vi "LogError.vi"(0 "Core In":refnum<class "Core.lvclass">, 11 "Error In":errorcluster {"Code" format="%.0x"}) -> (4 "Core Out":refnum<class "Core.lvclass">, 15 "Error Out":errorcluster {"Code" format="%.0x"})   [LabVIEW 2020, in "Core.lvlib" / "Core.lvclass"]
doc: "Logs error information from general error cluster and handles error codes based on the following conditions:\n- General errors (500,000 to 510,000)\n- Critical errors (510,001 to 520,000)\n- Fatal errors (520,001 to 530,000)"
uses:
  Core.lvclass
  Core.lvclass/Core.ctl
panel:
  # "/* Inputs */"
  # "/* Locals */"
  # "/* Outputs */"
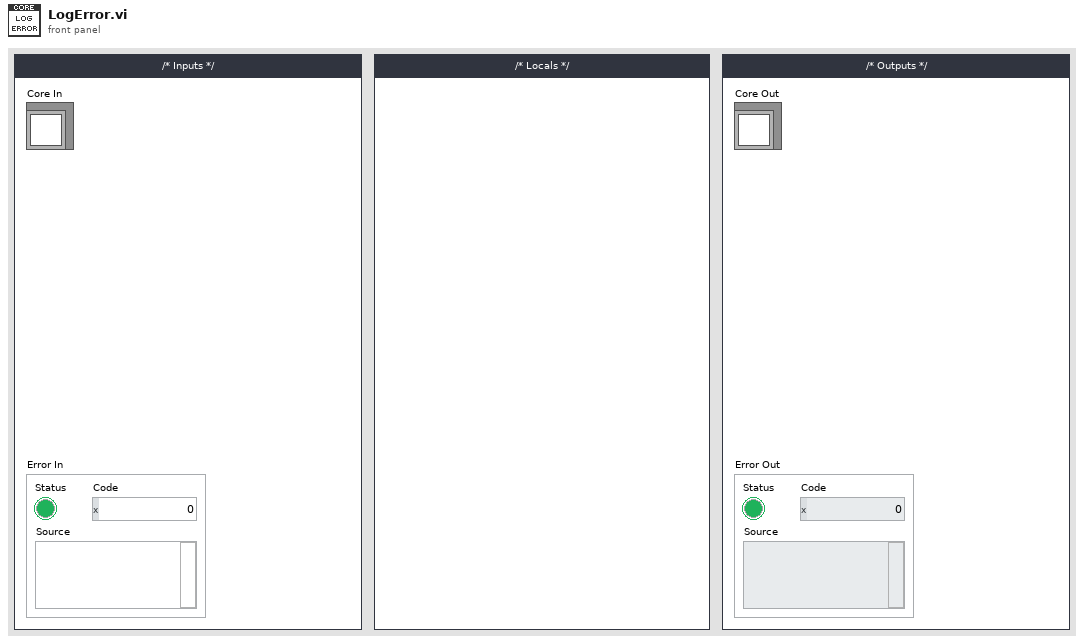
[diagram p1: front panel]
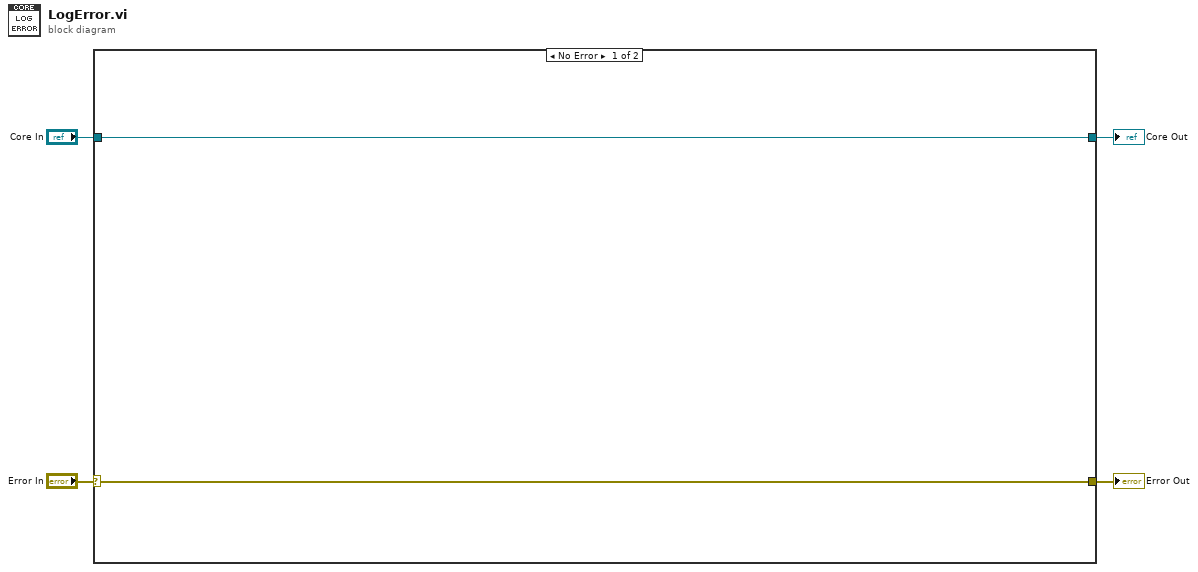
[diagram p0: block diagram]
diagram:
  n1 = case shown="No Error" "Error In" {
    selector: "Error In" -> [w6 w7]
    tunnel: [w6 w7] -> w3
    tunnel: "Core In" -> [w5 w8]
    tunnel: [w5 w8] -> w1
    frame No Error {
    }
    frame Error {
    }
  }
  "Core Out" <- w1
  "Error Out" <- w3
